vi "Pass Tuple Argument.vi"() -> ()   [LabVIEW 2019, in "OPI.lvclass"]
uses:
  OPI.lvclass
  Typedefs/Cmd Line Mode.ctl
  Get Return/Get Return - Pythonic.vi
  To Pythonic/To Pythonic - Boolean.vi
  To Pythonic/To Pythonic - Integer.vi
  To Pythonic/To Pythonic - Float.vi
  To Pythonic/To Pythonic - Tuple.vi
panel:
  out "Output Tuple":string
  out "Input Tuple":string
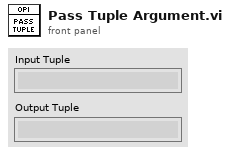
[diagram p1: front panel]
types:
  T1 = typedef "OPI.lvclass/Cmd Line Mode.ctl" = enum16{"Debug", "Hidden"}
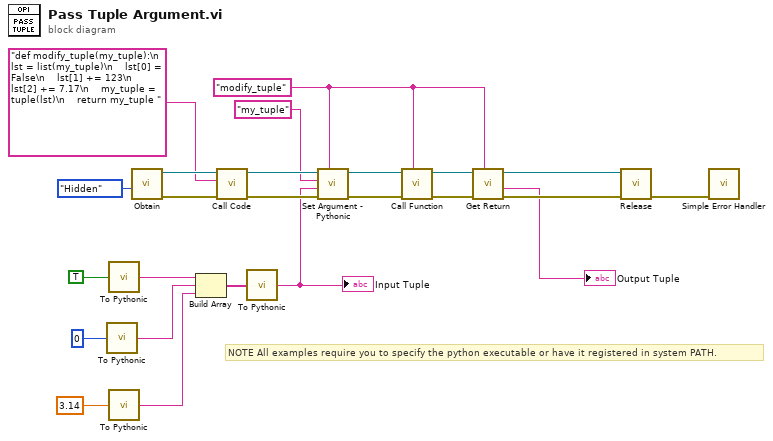
[diagram p0: block diagram]
diagram:
  w13 = "modify_tuple" ("Function")
  # "NOTE All examples require you to specify the python executable or have it registered in system PATH."
  n1 = call-poly "To Pythonic.vi"("Integer"=i64 0) -> ("Pythonic Value"=w4:string)  [unwired: 4 in]
  n2 = call-poly "To Pythonic.vi"("Boolean"=TRUE) -> ("Pythonic Value"=w5:string)  [unwired: 4 in]
  n3 = call-poly "To Pythonic.vi"("Float"=3.14) -> ("Pythonic Value"=w3:string)  [unwired: 4 in]
  n4 = call "Obtain.vi"("Cmd Line Mode (Hidden)"=Cmd_Line_Mode."Hidden") -> ("Error Out"=w23:errorcluster, "OPI Ref"=w24:refnum<data-value>)  [unwired: 9 in]
  n5 = Build Array(w5, w4, w3) -> (w2:string[])
  n6 = call "Call Code.vi"("Error In"=w23, "Pythonic Code"="def modify_tuple(my_tuple):\n    lst = list(my_tuple)\n    lst[0] = False\n    lst[1] += 123\n    lst[2] += 7.17\n    my_tuple = tuple(lst)\n    return my_tuple ", "OPI Ref"=w24) -> ("Error Out"=w10:errorcluster, "OPI Ref"=w14:refnum<data-value>)  [unwired: 7 in]
  n7 = call-poly "To Pythonic.vi"("Pythonic Values"=w2) -> ("Tuple"=w1:string)  [unwired: 4 in]
  "Input Tuple" <- w1
  n8 = call "Set Argument - Pythonic.vi"("Function Name"=w13, "Error In"=w10, "Pythonic Value"=w1, "Argument"="my_tuple" ("Function"), "OPI Ref"=w14) -> ("Error Out"=w11:errorcluster, "OPI Ref"=w12:refnum<data-value>)  [unwired: 5 in]
  n9 = call "Call Function.vi"("Function Name"=w13, "Error In"=w11, "OPI Ref"=w12) -> ("Error Out"=w18:errorcluster, "OPI Ref"=w19:refnum<data-value>)  [unwired: 7 in]
  n10 = call-poly "Get Return.vi"("Function Name"=w13, "Error In"=w18, "OPI Ref"=w19) -> ("Error Out"=w17:errorcluster, "Pythonic Return Value"=→"Output Tuple":string, "OPI Ref"=w21:refnum<data-value>)  [unwired: 6 in]
  n11 = call "Release.vi"("Error In"=w17, "OPI Ref"=w21) -> ("Error Out"=w16:errorcluster)  [unwired: 9 in]
  n12 = call <vilib>:"Simple Error Handler.vi"("error in (no error)"=w16) -> ()  [unwired: 4 in, 5 out]
